vi "Min Read Array.vi"(8 "error in":errorcluster, 11 "Min Voltage Limit in":refnum<class "Voltage Limit.lvclass">) -> (0 "error out":errorcluster, 1 "Changed or First Call?":bool, 2 "Voltage Min SP":dbl[](array[numeric]), 3 "Min Voltage Limit out":refnum<class "Voltage Limit.lvclass">)   [LabVIEW 2023, in "Voltage Limit.lvclass"]
uses:
  Voltage Limit.lvclass
  Voltage Limit.lvclass/Voltage Limit.ctl
  Parents/Limit/Limit.lvclass
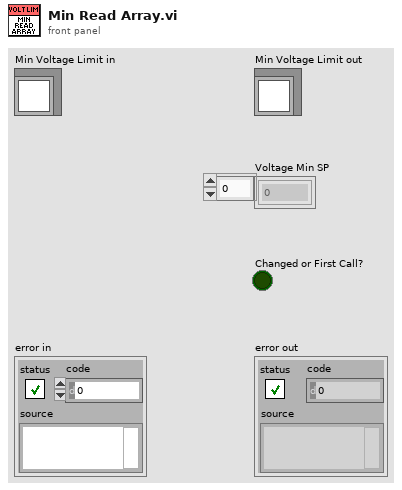
[diagram p1: front panel]
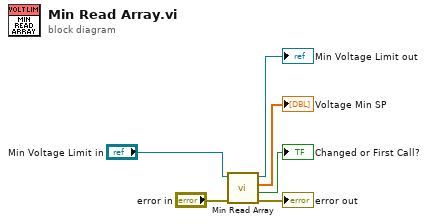
[diagram p0: block diagram]
diagram:
  n1 = call-parent "Min Read Array.vi"("error in"="error in", "Min Limit in"="Min Voltage Limit in") -> ("error out"=→"error out":errorcluster, "Changed or First Call?"=→"Changed or First Call?":bool, "Current Min SP"=→"Voltage Min SP":dbl[], "Min Limit out"=→"Min Voltage Limit out":refnum<class "Voltage Limit.lvclass">)  [unwired: 6 in]
